vi "Optimize Search.vi"(8 "Error In":errorcluster, 11 "Tree Manager":refnum<data-value>) -> (0 "Error Out":errorcluster, 3 "Tree Manager":refnum<data-value>)   [LabVIEW 2017, in "Tree API.lvlib" / "Tree.lvclass"]
doc: "Optimize search by looking at the whole Tree structure and creating a look-up table of search paths to all Trees. This is analogous to indexing a database."
uses:
  Tree.lvclass
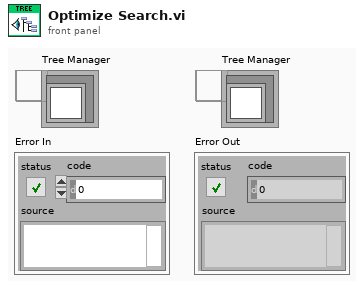
[diagram p1: front panel]
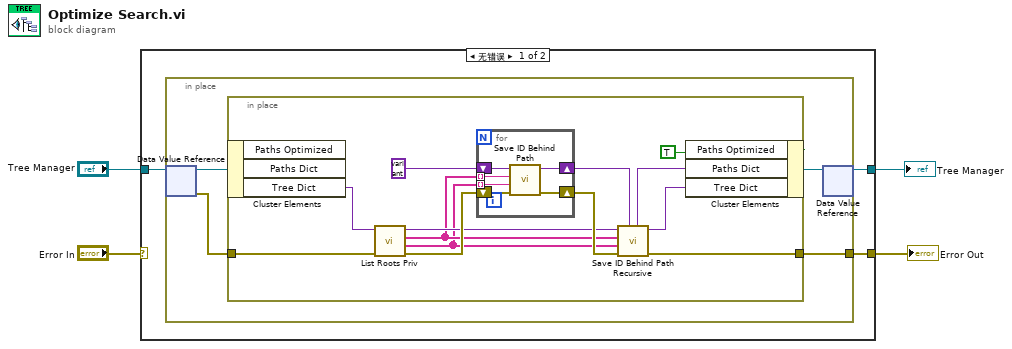
[diagram p0: block diagram]
diagram:
  n1 = case shown="无错误" "Error In" {
    selector: "Error In" -> [_ w31]
    tunnel: "Tree Manager" -> [w7 w32]
    tunnel: [w6 w32] -> w3
    tunnel: [w5 w31] -> w1
    frame No Error {
      n2 = in-place {
        in-place-border: [w8] -> w5
        n3 = in-place-dvr #1(w7) -> (w11:refnum<class "Tree.lvclass">, w9:errorcluster)
        n4 = in-place {
          in-place-border: w9 -> [w21]
          in-place-border: [w15] -> w8
          n5 = in-place-cluster #2(w11) -> ("Tree Dict"=w24:variant)  [unwired: 2 out]
          n6 = call "List Roots Priv.vi"("error in"=w21, "Tree Dict"=w24) -> ("error out"=w22:errorcluster, "Root Names"=w12:string[], "Root IDs"=w13:string[], "Tree Dict"=w18:variant)  [unwired: 6 in]
          n7 = for {
            shift-right: [w27] -> w17
            shift-left: variant -> [w30]
            shift-right: [w28] -> w20
            shift-left: w22 -> [w29]
            tunnel: w13 -> [w26] mode=indexing
            tunnel: w12 -> [w25] mode=indexing
            n8 = call "Save ID Behind Path.vi"("Error In"=w29, "Paths"=w25, "IDs"=w26, "Paths Dict"=w30) -> ("Error Out"=w28:errorcluster, "Paths Dict"=w27:variant)  [unwired: 6 in]
          }
          n9 = call "Save ID Behind Path Recursive.vi"("Paths Dict In"=w17, "Error In"=w20, "Parent Path"=w12, "Parent IDs"=w13, "Tree Dict In"=w18) -> ("Error Out"=w15:errorcluster, "Tree Dict Out"=w16:variant, "Paths Dict Out"=w14:variant)  [unwired: 4 in]
          n10 = in-place-cluster #2("Paths Optimized"=TRUE, "Paths Dict"=w14, "Tree Dict"=w16) -> (w10:refnum<class "Tree.lvclass">)
        }
        n11 = in-place-dvr #1(w10) -> (w6:refnum<data-value>)  [unwired: 1 out]
      }
    }
    frame Error {
    }
  }
  "Tree Manager" <- w3
  "Error Out" <- w1
